vi "Filter FFT (SubVI).vi"(10 "取FFT的前面點數":i8=20, 11 "Input":dbl[](array[numeric])) -> (3 "Output":dbl[](array[numeric]))   [LabVIEW 2019]
uses:
  <vilib>/Analysis/NI_AALPro.lvlib
  <vilib>/Analysis/2dsp.llb/Real FFT.vi
  <vilib>/Analysis/2dsp.llb/Inverse Real FFT.vi
panel:
  out "error out":errorcluster
  in  "error in (no error)":errorcluster
  out "FFT {X}":cdb[](array[numeric])
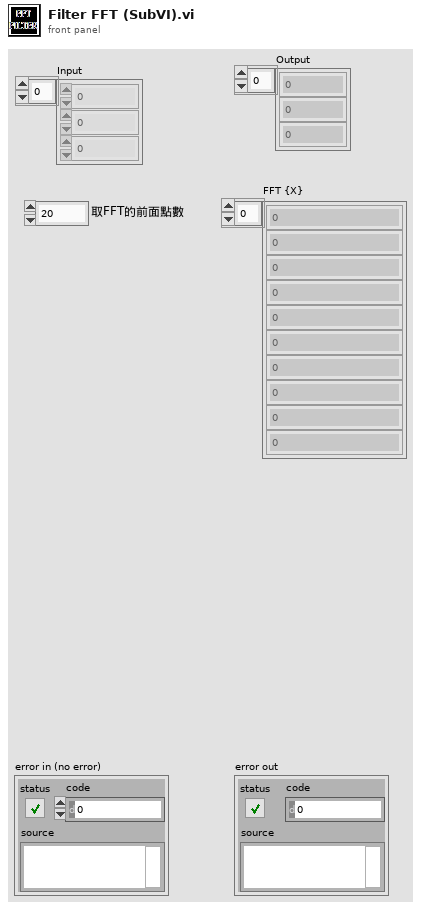
[diagram p1: front panel]
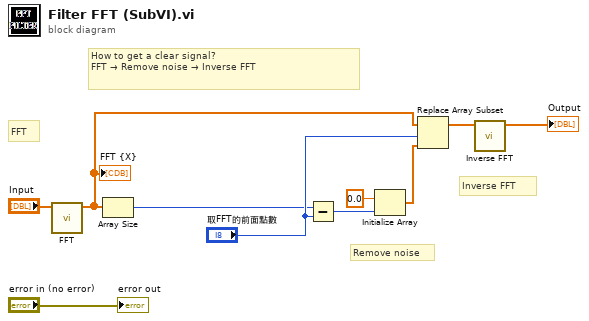
[diagram p0: block diagram]
diagram:
  # "Inverse FFT"
  # "Remove noise"
  # "FFT"
  # "How to get a clear signal? \nFFT → Remove noise → Inverse FFT"
  n1 = call-poly <vilib>:"FFT.vi"("X"="Input") -> ("FFT {X}"=w4:cdb[])  [unwired: 9 in, 1 out]
  "FFT {X}" <- w4
  n2 = Array Size(array=w4) -> (size(s)=w2:i32)
  n3 = Subtract(x=w2, y="取FFT的前面點數") -> (x-y=w3:i32)
  n4 = Initialize Array(0.0 ("element"), w3) -> (w5:dbl[])
  n5 = Replace Array Subset(array=w4, new element=w5, index="取FFT的前面點數") -> (w7:cdb[])
  n6 = call-poly <vilib>:"Inverse FFT.vi"("FFT {X}"=w7) -> ("X"=→"Output":dbl[])  [unwired: 9 in, 1 out]
  "error out" <- "error in (no error)"
